vi "TTA_MATLAB_Tile_Set_PA_Control.vi"(0 "Channels":string[](array[combo]), 1 "OutPower":i32, 2 "InPower":i32, 5 "Temp":i32, 7 "Current":i32, 11 "error in":errorcluster) -> (4 "Success":bool, 6 "TileSuccessComm":bool[](array[boolean]), 8 "TileSuccessOp":bool[](array[boolean]), 15 "error out":errorcluster)   [LabVIEW 2016]
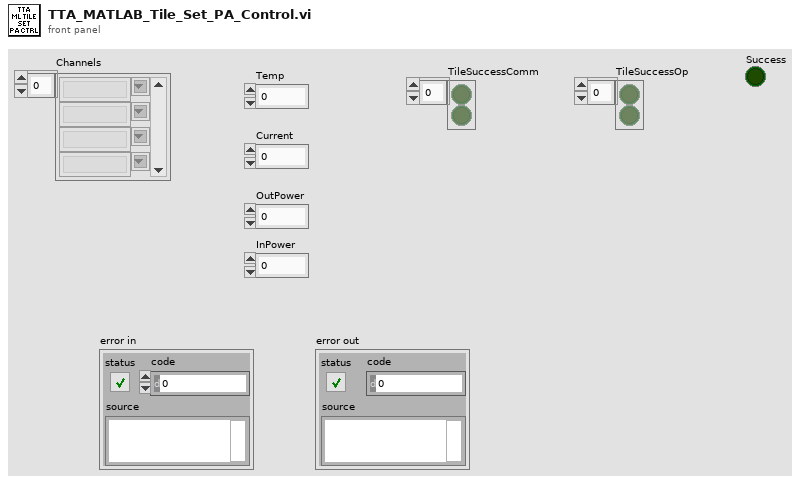
[diagram p1: front panel]
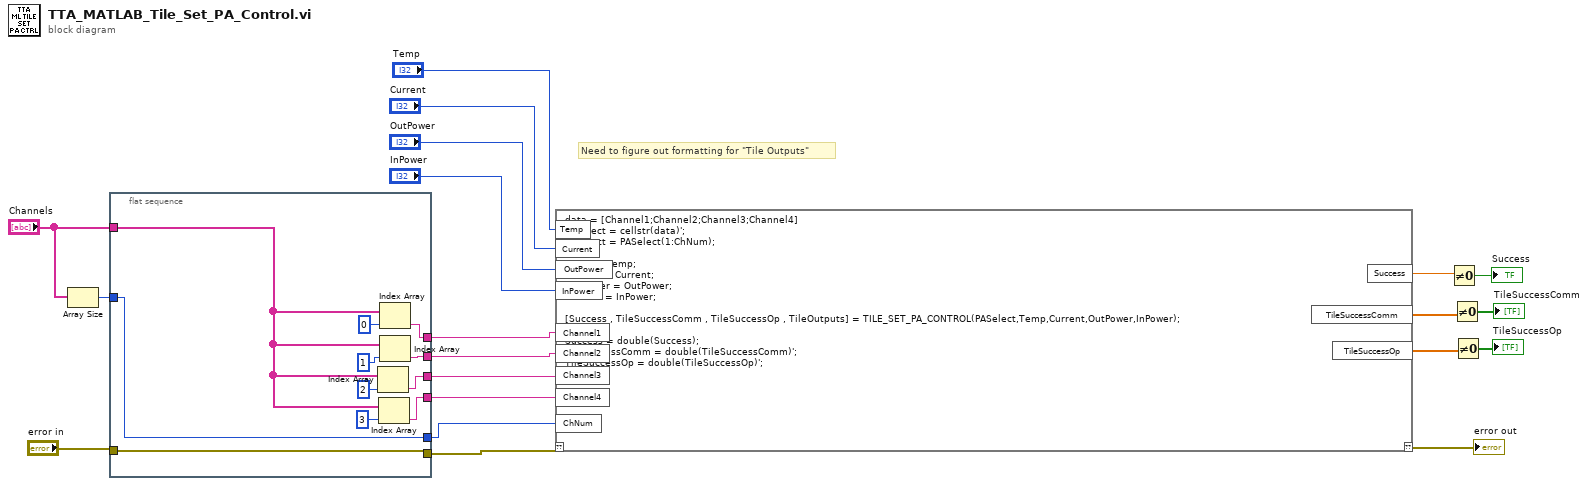
[diagram p0: block diagram]
diagram:
  # "Need to figure out formatting for \"Tile Outputs\""
  n1 = Array Size(array="Channels") -> (size(s)=w8:i32)
  n2 = flat-sequence {
    tunnel: "error in" -> [w31]
    tunnel: [w30] -> w5
    tunnel: w8 -> [w24]
    tunnel: [w31] -> w6
    tunnel: "Channels" -> [w23]
    tunnel: [w27] -> w4
    tunnel: [w25] -> w3
    tunnel: [w24] -> w1
    tunnel: [w21] -> w2
    frame #0 {
      n3 = Index Array(array=w23, index=2) -> (element=w25:string)
      n4 = Index Array(array=w23, index=3) -> (element=w21:string)
      n5 = Index Array(array=w23, index=0) -> (element=w30:string)
      n6 = Index Array(array=w23, index=1) -> (element=w27:string)
    }
  }
  n7 = script code="data = [Channel1;Channel2;Channel3;Channel4]\nPASelect = cellstr(data)';\nPASelect = PASelect(1:ChNum);\n\nTemp = Temp;\nCurrent = Current;\nOutPower = OutPower;\nInPower = InPower;\n\n[Success , TileSuccessComm , TileSuccessOp , TileOutputs] = TILE_SET_PA_CONTROL(PASelect,Temp,Current,OutPower,InPower);\n\nSuccess = double(Success);\nTileSuccessComm = double(TileSuccessComm)';\nTileSuccessOp = double(TileSuccessOp)';"("??"=w6, "Channel1"=w5, "Temp"="Temp", "Current"="Current", "OutPower"="OutPower", "InPower"="InPower", "Channel2"=w4, "Channel3"=w3, "Channel4"=w2, "ChNum"=w1) -> ("??"=→"error out":errorcluster, "Success"=w12:dbl, "TileSuccessComm"=w11:dbl[], "TileSuccessOp"=w10:dbl[])
  n8 = Not Equal To 0?(x=w12) -> (x != 0?=→"Success":bool)
  n9 = Not Equal To 0?(x=w11) -> (x != 0?=→"TileSuccessComm":bool[])
  n10 = Not Equal To 0?(x=w10) -> (x != 0?=→"TileSuccessOp":bool[])
